vi "global_FT Handle.vi"() -> ()   [LabVIEW 2019]
panel:
  out "FT_Handle":u32
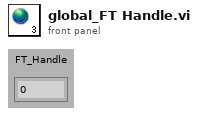
[diagram p1: front panel]
diagram:
